vi "Create Temp Config File.vi"(0 "Config File Path":path, 5 "Paths to Filter out":refnum<class "Path.lvclass">[](array[class]), 11 "error in":errorcluster) -> (4 "Temp Config File Path":path, 15 "error out":errorcluster)   [LabVIEW 2023, in "RFFixtureCharact.Public.lvlib"]
uses:
  RFFixtureCharact.Public.lvlib
  Common/Base Classes/Path/Path.lvclass
  <vilib>/Utility/file.llb/Read Delimited Spreadsheet (string).vi
  <vilib>/Utility/file.llb/Write Delimited Spreadsheet (string).vi
  Common/RFCalAndFixtureCharact.Common.lvlib
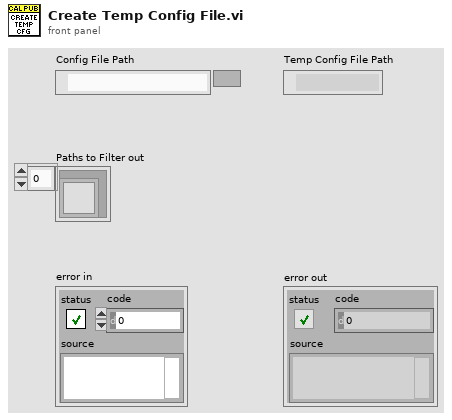
[diagram p1: front panel]
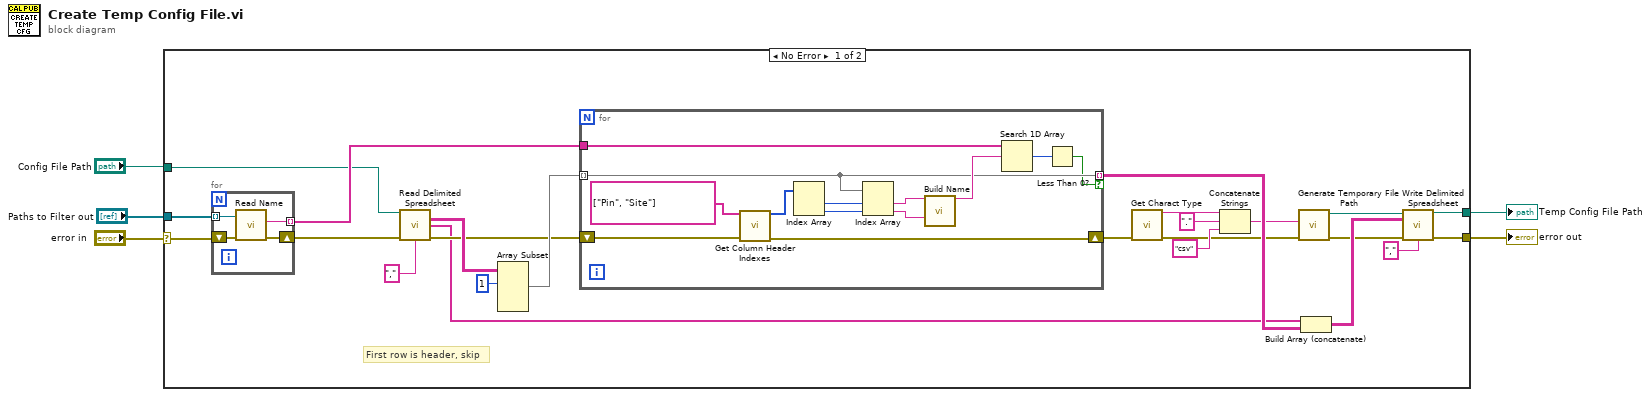
[diagram p0: block diagram]
diagram:
  n1 = case shown="No Error" "error in" {
    selector: "error in" -> [w16 w47]
    tunnel: [w22 w47] -> w4
    tunnel: "Config File Path" -> [w12 _]
    tunnel: "Paths to Filter out" -> [w25 _]
    tunnel: [w20 _] -> w1
    frame No Error {
      # "First row is header, skip"
      n2 = for {
        tunnel: w25 -> [w33] mode=indexing
        tunnel: [w32] -> w13 mode=indexing
        shift-right: [w30] -> w15
        shift-left: w16 -> [w31]
        n3 = call-dynamic "Read Name.vi"("error in (no error)"=w31, "Path in"=w33) -> ("error out"=w30:errorcluster, "Name"=w32:string)  [unwired: 7 in, 1 out]
      }
      n4 = call-poly <vilib>:"Read Delimited Spreadsheet.vi"("file path (dialog if empty)"=w12, "error in (no error)"=w15, "delimiter (\\t)"="," ("delimiter (\\t)")) -> ("all rows"=w28:string[][], "first row"=w14:string[], "error out"=w23:errorcluster)  [unwired: 7 in, 3 out]
      n5 = Array Subset(array=w28, index (row)=1 ("index")) -> (w26:string[][])  [unwired: 3 in]
      n6 = for {
        tunnel: w26 -> [w39] mode=indexing
        tunnel: w13 -> [w41]
        tunnel: [w39] -> w24 mode=indexing if=w37
        shift-right: [w35] -> w8
        shift-left: w23 -> [w36]
        n7 = call "Get Column Header Indexes.vi"("Column Header Names"=string[] ["Pin", "Site"], "error in"=w36) -> ("Column Header Indices"=w45:i32[], "error out"=w35:errorcluster)  [unwired: 11 in, 1 out]
        n8 = Index Array(array=w45) -> (element #1=w44:i32, element #2=w43:i32)  [unwired: 2 in]
        n9 = Index Array(array=w39, index #1=w44, index #2=w43) -> (element #1=w42:string, element #2=w34:string)
        n10 = call "Build Name.vi"("Pin"=w42, "Site"=w34) -> ("Path name"=w40:string)  [unwired: 13 in]
        n11 = Search 1D Array(1D array=w41, element=w40) -> (index of element=w38:i32)  [unwired: 1 in]
        n12 = Less Than 0?(x=w38) -> (x < 0?=w37:bool)
      }
      n13 = call "Get Charact Type.vi"("error in (no error)"=w8) -> ("Charact type"=w6:string, "error out"=w7:errorcluster)  [unwired: 13 in]
      n14 = Concatenate Strings(w6, "." ("string"), "csv" ("string")) -> (w11:string)
      n15 = call <vilib>:"Generate Temporary File Path.vi"("error in (no error)"=w7, "Temporary File Extension (tmp)"=w11) -> ("error out"=w19:errorcluster, "Unique Temporary File Path"=w18:path)  [unwired: 8 in]
      n16 = Build Array (concatenate)(w14, w24) -> (w21:string[][])
      n17 = call-poly <vilib>:"Write Delimited Spreadsheet.vi"("file path (dialog if empty)"=w18, "2D data"=w21, "error in (no error)"=w19, "delimiter (\\t)"="," ("delimiter (\\t)")) -> ("new file path (Not A Path if cancelled)"=w20:path, "error out"=w22:errorcluster)  [unwired: 10 in]
    }
    frame Error {
    }
  }
  "error out" <- w4
  "Temp Config File Path" <- w1
